vi "Read Language.vi"(8 "error in (no error)":errorcluster, 11 "Prooduct Actor in":refnum<class "Prooduct Actor.lvclass">) -> (0 "error out":errorcluster, 2 "Language":T1, 3 "Prooduct Actor out":refnum<class "Prooduct Actor.lvclass">)   [LabVIEW 2020, in "Prooduct Actor.lvlib" / "Prooduct Actor.lvclass"]
uses:
  Prooduct Actor.lvclass
  Controls/Language Enum.ctl
  Prooduct Actor.lvclass/Prooduct Actor.ctl
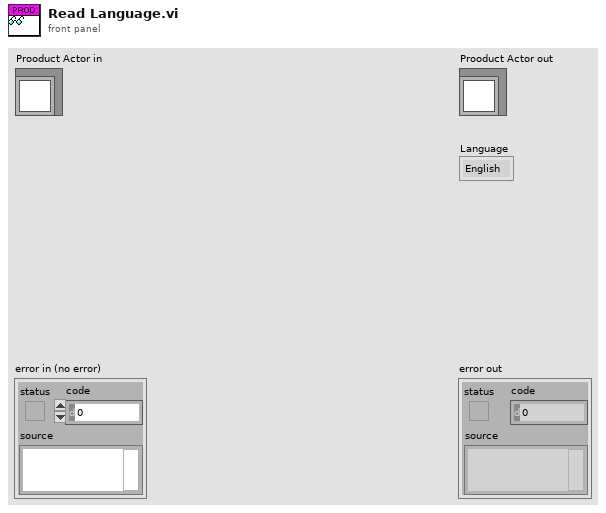
[diagram p1: front panel]
types:
  T1 = typedef "Language Enum.ctl" = enum16{"English", "Español", "Français"}
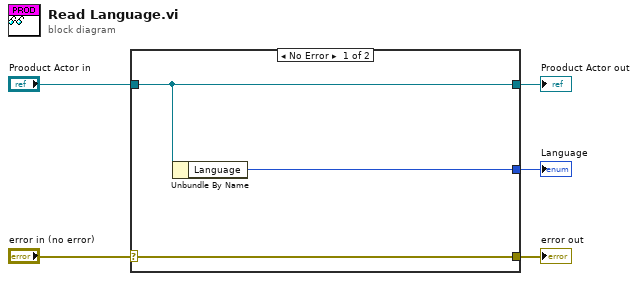
[diagram p0: block diagram]
diagram:
  n1 = case shown="No Error" "error in (no error)" {
    selector: "error in (no error)" -> [w8 w9]
    tunnel: [w8 w9] -> w4
    tunnel: [w7 w10] -> w2
    tunnel: "Prooduct Actor in" -> [w7 w10]
    tunnel: [w6 _] -> w1
    frame No Error {
      n2 = Unbundle By Name(w7) -> ("Language"=w6:T1)
    }
    frame Error {
    }
  }
  "error out" <- w4
  "Prooduct Actor out" <- w2
  "Language" <- w1
